vi "random_bit.vi"(1 "Количество бит":i32=8) -> (0 "Биты на выходе 1":dbl[](array[numeric]))   [LabVIEW 2013]
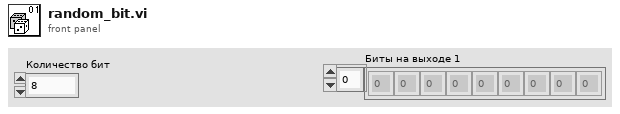
[diagram p1: front panel]
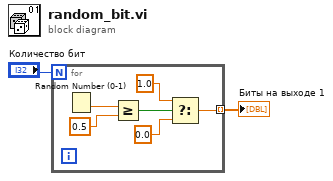
[diagram p0: block diagram]
diagram:
  n1 = for {
    N: "Количество бит" -> [_]
    tunnel: [w3] -> w1 mode=indexing
    n2 = Random Number (0-1)() -> (number: 0 to 1=w8:dbl)
    n3 = Greater Or Equal?(x=w8, y=0.5) -> (x >= y?=w6:bool)
    n4 = Select(t=1.0, s=w6, f=0.0) -> (s? t:f=w3:dbl)
  }
  "Биты на выходе 1" <- w1
